vi "DualDigitalOscilloscope .vi"() -> ()   [LabVIEW 2014]
doc: "This is a modification of the previous oscilliscope. This VI acts as a digital oscilliscope with 2 different inputs. Voltage signals applied to ai0 and ai1 on the daq can be plotted on the oscilliscope. The signals require a TTL trigger to view a stationary waveform."
panel:
  out "Waveform Graph":dynamicdata(graph)=[{"t0"=timestamp(3496345101.638286 s since 1904-01-01), "dt"=0.001, "Y"=array[500 elements], "attributes"=variant("NI_ChannelName"=variant(string "Voltage 1"), "NI_UnitDescription"=variant(string "Volts"))}, {"t0"=timestamp(3496345101.638298 s since 1904-01-01), "dt"=0.001, "Y"=array[500 elements], "attributes"=variant("NI_ChannelName"=variant(string "Voltage 2"), "NI_UnitDescription"=variant(string "Volts"))}]
  out "error out":errorcluster
  in  "Digitizing Parameters":T1={"Number of Samples"=500.0, "Sampling Frequency"=1000.0}
  in  "stop":bool
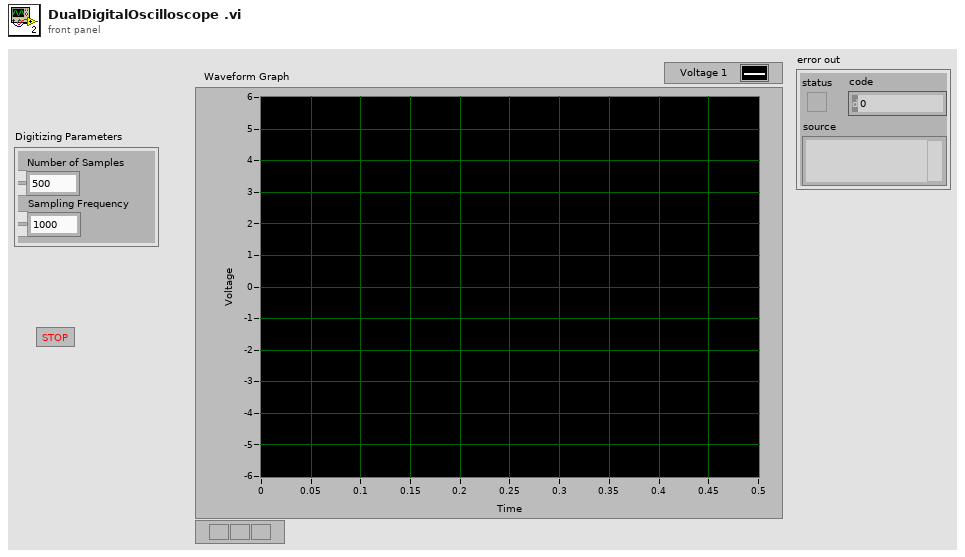
[diagram p1: front panel]
types:
  T1 = cluster{"Number of Samples":dbl, "Sampling Frequency":dbl}
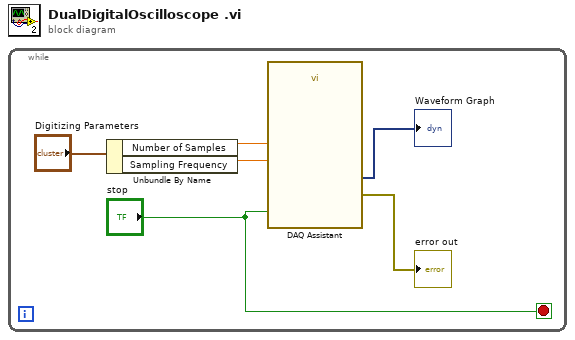
[diagram p0: block diagram]
diagram:
  n1 = while {
    stop <- "stop" stop-if-true
    n2 = Unbundle By Name("Digitizing Parameters") -> ("Number of Samples"=w5:dbl, "Sampling Frequency"=w4:dbl)
    n3 = call "DAQ Assistant"("rate"=w4, "number of samples"=w5, "stop (T)"="stop") -> ("data"=→"Waveform Graph":dynamicdata, "error out"=→"error out":errorcluster)  [unwired: 14 in, 1 out]
  }
